vi "Main.vi"() -> ()   [LabVIEW 2018, in "MQTT_Singleton.lvlib"]
doc: "This template is based off of the Queued Message Handler design pattern and the Queued Message Handler project template that ships with LabVIEW.\n\nThe main difference is that the queue is private to this module and communication between modules is performed via Broadcast and Request events.\n\nRequest events are wrapped in public API methods and are handled in the Event Handling Loop (EHL) of this VI. Any module can register for Broadcast events sent by this module. The EHL generates messages based on user interface actions.\n\nThe Message Handling Loop (MHL) processes messages generated by the EHL, or by other messages. The messages are string values, so new messages can be added easily to the Message Cases case structure in the MHL. Each message cluster can also provide an optional value for Message Data, which is a variant that can be converted to whatever message-specific data is required.\n_____\nBased on Delacor QMH Project Template 4.1.0.59."
uses:
  MQTT_Singleton.lvlib
  <vilib>/Delacor/Delacor QMH/Libraries/Module Admin_class/Delacor_lib_QMH_Module Admin.lvclass
  Module Data--cluster.ctl
  LVMQTT-master/Controls/Connection_Return_Codes.ctl
  LVMQTT-master/Controls/QoS.ctl
  LVMQTT-master/Controls/DUP_Flag.ctl
  LVMQTT-master/Controls/Retain_Flag.ctl
  Stop Argument--cluster.ctl
  <vilib>/Delacor/Delacor QMH/Libraries/Module Admin_class/Delacor_lib_QMH_Module Admin.lvclass/Delacor_lib_QMH_Module Admin.ctl
  Connect Argument--cluster.ctl
  Publish Argument--cluster.ctl
  Subscribe Argument--cluster.ctl
  Disconnect Argument--cluster.ctl
  <vilib>/Utility/miscctls.llb/LVPointTypeDef.ctl
  LVMQTT-master/Controls/Connect_Flags.ctl
  <vilib>/Delacor/Delacor QMH/Libraries/Module Admin_class/Delacor_lib_QMH_Get External Launch.vi
  HB.vi
  <vilib>/Delacor/Delacor QMH/Libraries/Message Queue_class/Delacor_lib_QMH_Enqueue Message (Single).vi
  <vilib>/Utility/error.llb/Error Cluster From Error Code.vi
  <vilib>/ErrorRing/Error Ring.xnode
  <vilib>/Delacor/Delacor QMH/Libraries/Message Queue_class/Delacor_lib_QMH_Message Queue.lvclass
  LVMQTT-master/MQTT_Functions.lvlib
  MQTT Messages.lvlib
panel:
  out "Publish Message":string
  out "Publish Topic":string
  out "HB RX Count":u32
  out "Subscribe Topic":string
  out "Rx Message":string
  out "Rx Topic Name":string
  out "Latency (ms)":u32
  out "ms":u32
  out "HB TX Count":u32
  out "Acknowledged":bool
  out "error out":errorcluster
  in  "Module Admin":refnum<class "Delacor_lib_QMH_Module Admin.lvclass">
  out "Status":string
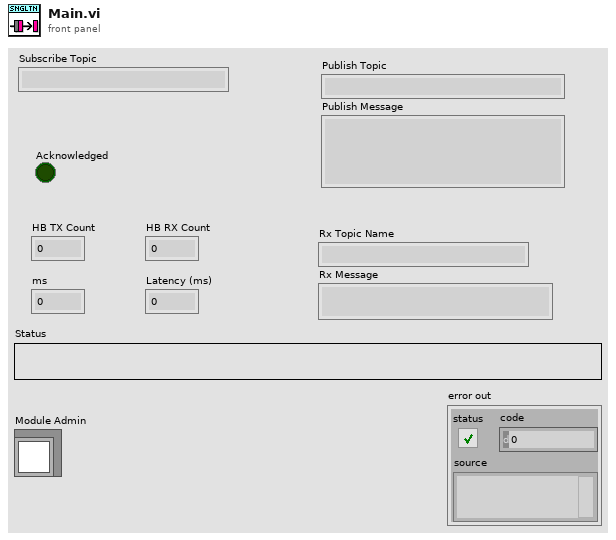
[diagram p1: front panel]
types:
  T1 = typedef "MQTT_Singleton.lvlib/Request Events--cluster.ctl" = cluster{"Stop Module":refnum<user-event>, "Show Panel":refnum<user-event>, "Hide Panel":refnum<user-event>, "Get Module Execution Status":refnum<user-event>, "Show Diagram":refnum<user-event>, "Connect":refnum<user-event>, "Publish":refnum<user-event>, "Subscribe":refnum<user-event>, "Disconnect":refnum<user-event>, "Start Listening":refnum<user-event>, "Stop Listening":refnum<user-event>, "Exit Listening":refnum<user-event>}
  T2 = typedef "MQTT_Singleton.lvlib/Module Data--cluster.ctl" = cluster{"Status":string, "connection ID out":refnum<k5>, "Connection Status":T3, "Connect Meta":cluster{"QoS":T4, "DUP":T5, "Retain":T6, "Keep Alive (sec)":u16}, "Message ID":u16, "Listening?":bool, "Default Topics":string[], "Broker IP":string, "Client ID":string}
  T3 = typedef "MQTT_Functions.lvlib/Connection_Return_Codes.ctl" = enum16{"Connection accepted", "Connection refused: unacceptable protocol version", "Connection refused: identifier rejected", "Connection refused: Server unavailable", "Connection refused: bad user name or password", "Connection refused: not authorized"}
  T4 = typedef "MQTT_Functions.lvlib/QoS.ctl" = enum8{"At most once", "At least once", "Exactly once", "Reserved"}
  T5 = typedef "MQTT_Functions.lvlib/DUP_Flag.ctl" = bool
  T6 = typedef "MQTT_Functions.lvlib/Retain_Flag.ctl" = bool
  T7 = enum32{"invalid lock state", "Not Locked", "Locked (No Password)", "Password-protected"}
  T8 = typedef "MQTT_Singleton.lvlib/Stop Argument--cluster.ctl" = cluster{"Origin":string, "Exit via Stop Module Req?":bool, "Wait for Module to stop?":bool}
  T9 = typedef "MQTT_Singleton.lvlib/Connect Argument--cluster.ctl" = cluster{"Broker IP":string, "ClientID":string}
  T10 = typedef "MQTT_Singleton.lvlib/Publish Argument--cluster.ctl" = cluster{"Topic":string, "Message":string}
  T11 = typedef "MQTT_Singleton.lvlib/Subscribe Argument--cluster.ctl" = cluster{"Topic":string}
  T12 = typedef "MQTT_Singleton.lvlib/Disconnect Argument--cluster.ctl" = cluster{"Disconnect?":bool}
  T13 = typedef "LVPointTypeDef.ctl" = cluster{"Horizontal":i16, "Vertical":i16}
  T14 = enum32{"Invalid", "Standard", "Closed", "Hidden", "Minimized", "Maximized"}
  T15 = cluster{"QoS":T4, "DUP":T5, "Retain":T6, "Keep Alive (sec)":u16}
  T16 = typedef "MQTT_Functions.lvlib/Connect_Flags.ctl" = cluster{"user name":bool, "password":bool, "will retain":bool, "will flag":bool, "clean session":bool, "reserved":bool, "will QoS":T4}
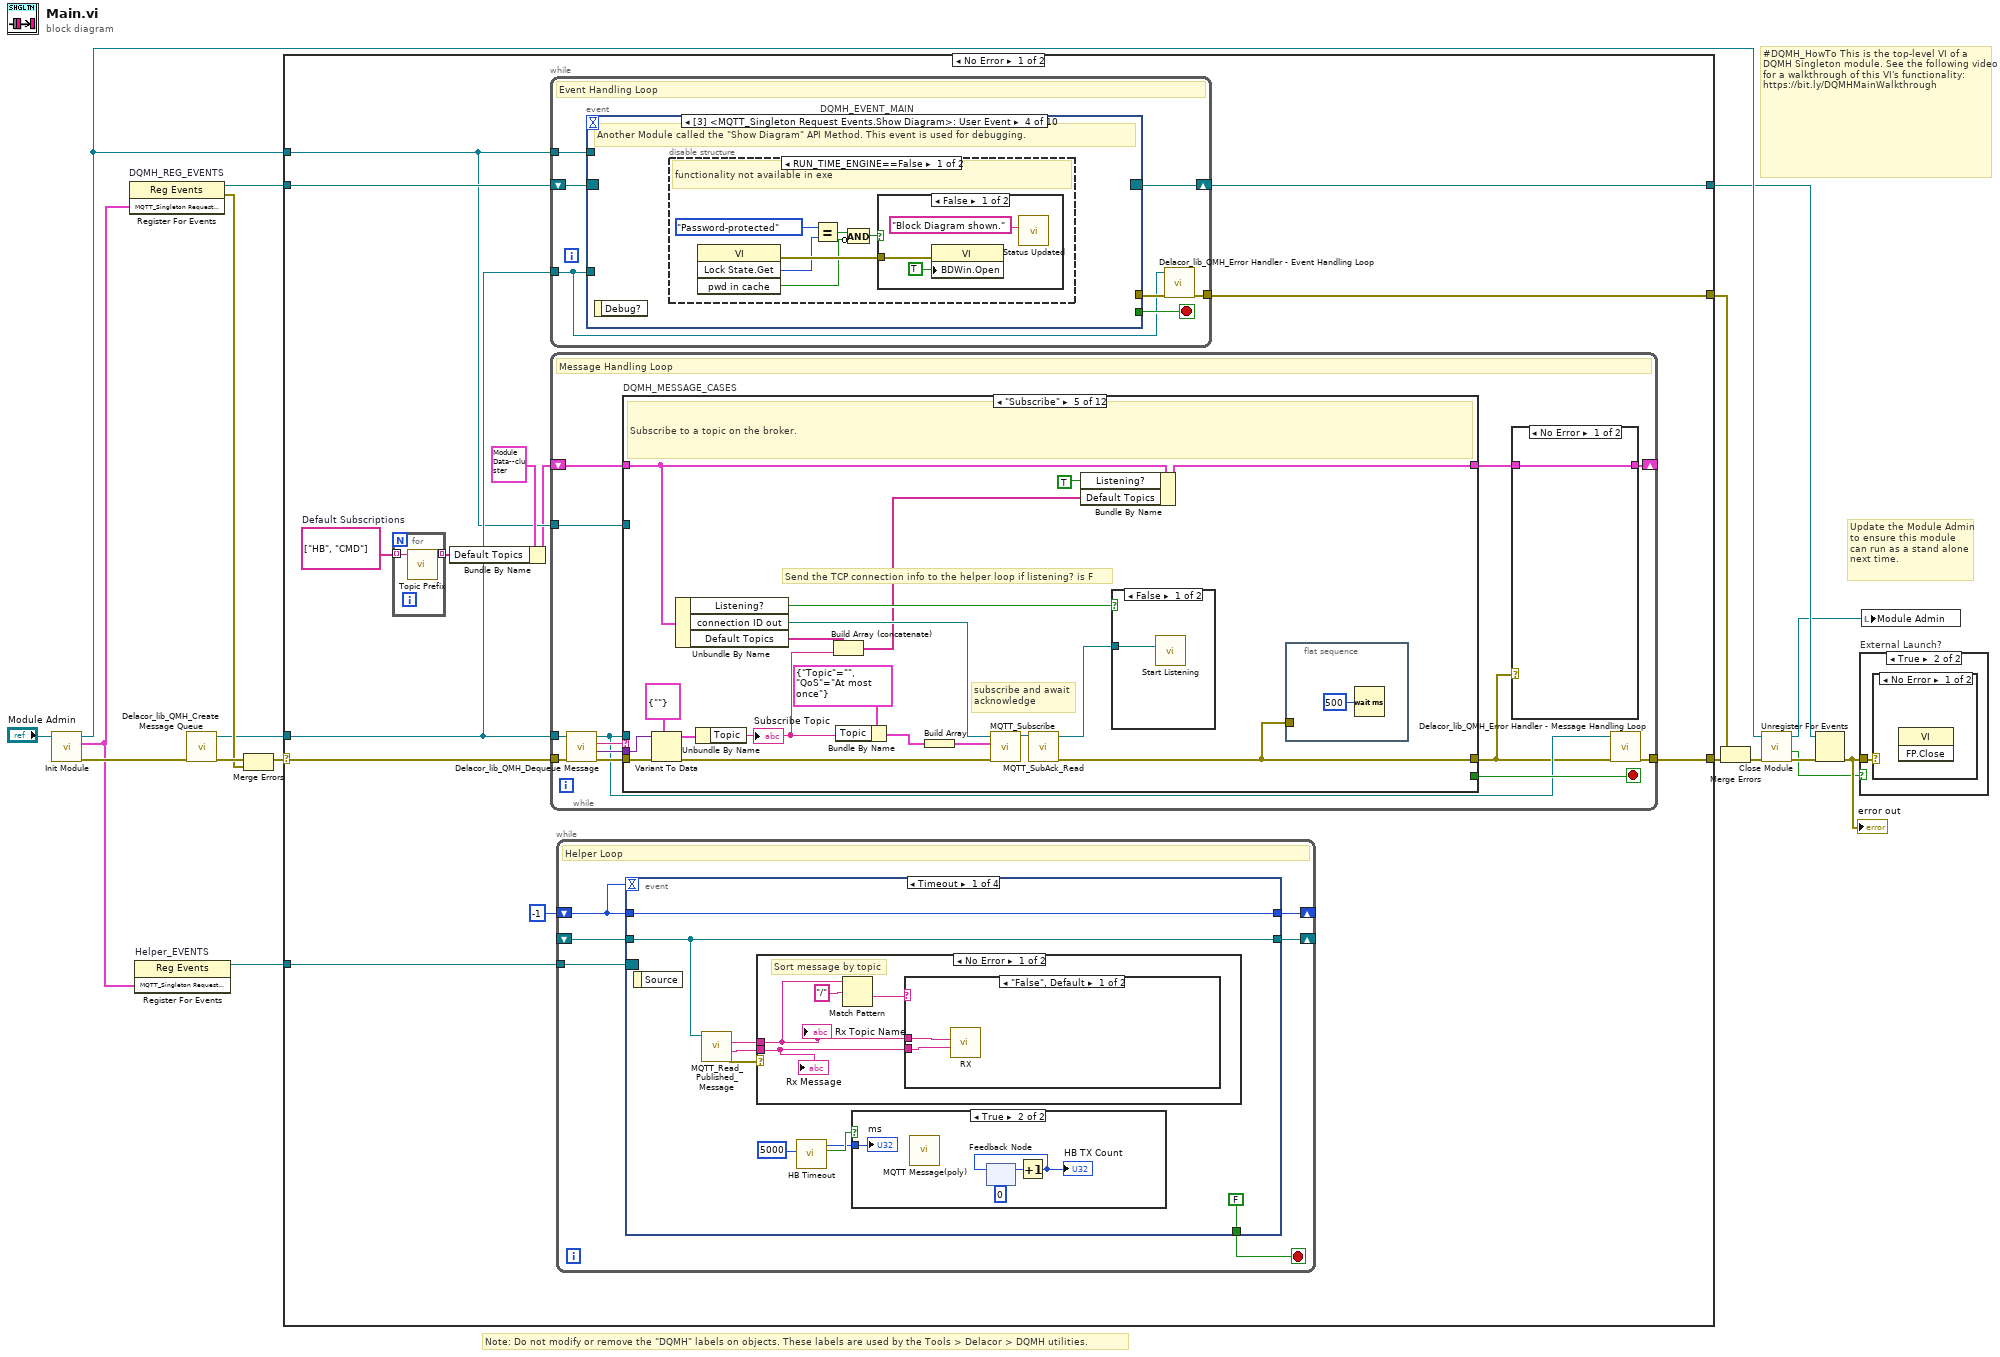
[diagram p0: block diagram]
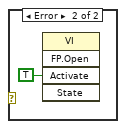
[diagram p3: hidden frame]
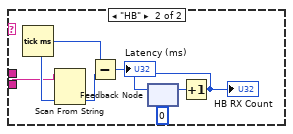
[diagram p5: hidden frame]
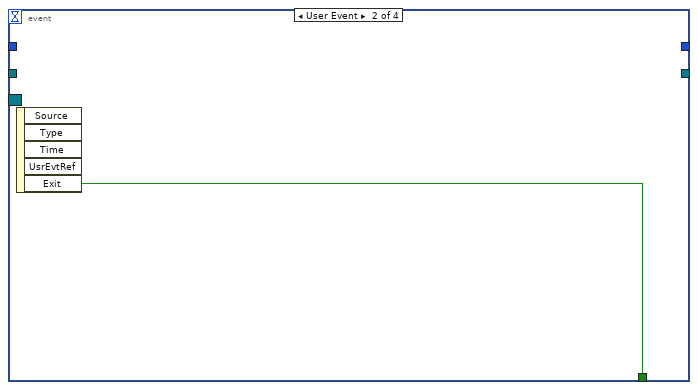
[diagram p7: hidden frame]
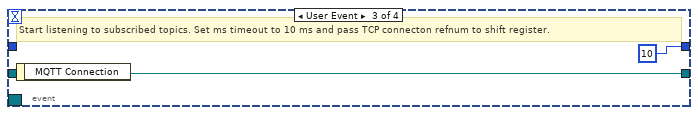
[diagram p8: hidden frame]
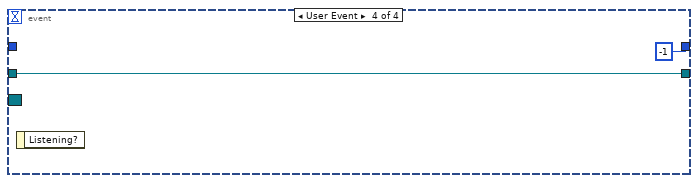
[diagram p9: hidden frame]
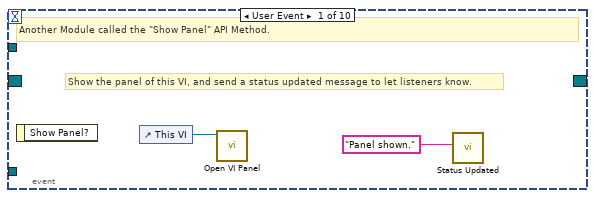
[diagram p10: hidden frame]
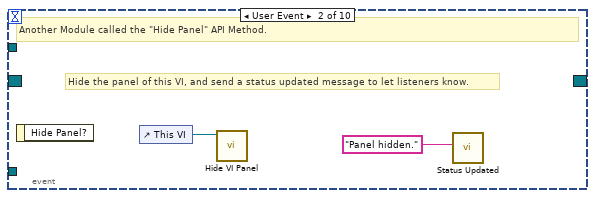
[diagram p11: hidden frame]
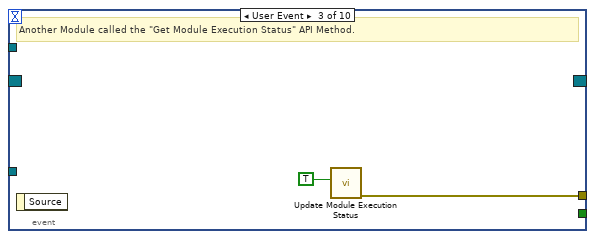
[diagram p12: hidden frame]
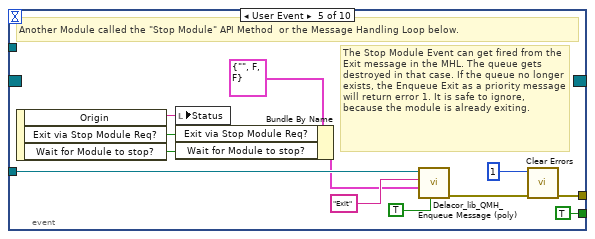
[diagram p15: hidden frame]
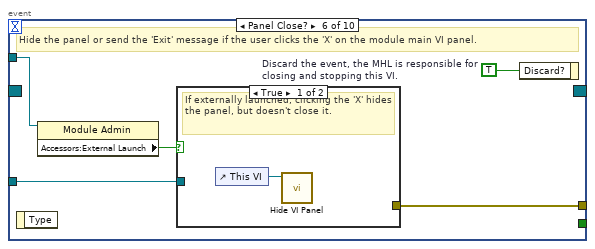
[diagram p16: hidden frame]
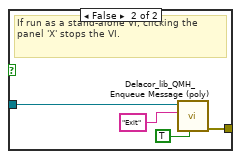
[diagram p17: hidden frame]
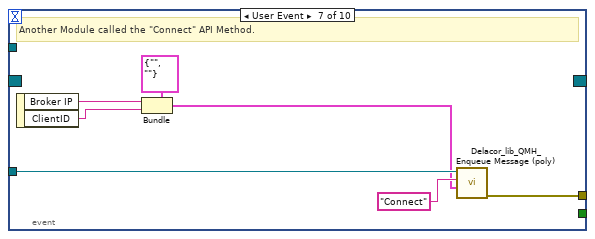
[diagram p18: hidden frame]
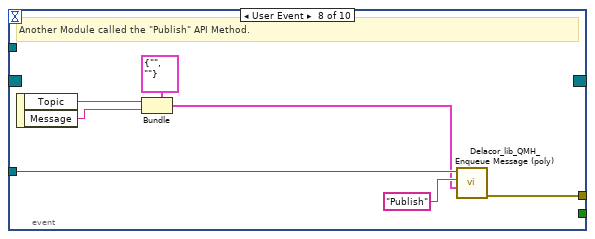
[diagram p19: hidden frame]
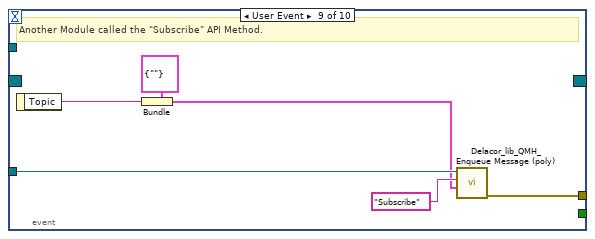
[diagram p20: hidden frame]
diagram:
  # "#DQMH_HowTo This is the top-level VI of a DQMH Singleton module. See the following video for a walkthrough of this VI's functionality: https://bit.ly/DQMHMainWalkthrough"
  # "Note: Do not modify or remove the \"DQMH\" labels on objects. These labels are used by the Tools > Delacor > DQMH utilities."
  # "Update the Module Admin to ensure this module can run as a stand alone next time."
  n1 = call "Init Module.vi"("Singleton Module Admin in"="Module Admin") -> ("error out"=w17:errorcluster, "MQTT_Singleton Request Events"=w2:T1, "Singleton Module Admin out"=w9:refnum<class "Delacor_lib_QMH_Module Admin.lvclass">)  [unwired: 8 in]
  n2 = register-events "DQMH_REG_EVENTS"(w2) -> (reference out=w7:refnum<event-registration>, error out=w10:errorcluster)  [unwired: 2 in]
  n3 = register-events "Helper_EVENTS"(w2) -> (reference out=w1:refnum<event-registration>)  [unwired: 2 in, 1 out]
  n4 = call <vilib>:"Delacor_lib_QMH_Create Message Queue.vi"("error in (no error)"=w17) -> ("error out"=w12:errorcluster, "Message Queue"=w6:refnum<class "Delacor_lib_QMH_Message Queue.lvclass">)  [unwired: 9 in]
  n5 = Merge Errors(w12, w10) -> (w11:errorcluster)
  n6 = case shown="No Error" w11 {
    selector: w11 -> [w29 w371]
    tunnel: [w31 w371] -> w18
    tunnel: [w28 w368] -> w8
    tunnel: w7 -> [w26 w368]
    tunnel: w6 -> [w25 _]
    tunnel: [w30 _] -> w15
    tunnel: w9 -> [w24 w364]
    tunnel: w1 -> [w22 _]
    frame No Error {
      w20 = string[] ["HB", "CMD"]  # Default Subscriptions
      n7 = for {
        tunnel: w20 -> [w33] mode=indexing
        tunnel: [w32] -> w19 mode=indexing
        n8 = call "Topic Prefix.vi"("Topic"=w33) -> ("Topic"=w32:string)  [unwired: 9 in, 1 out]
      }
      n9 = Bundle By Name(cluster=T2 {"Status"="", "connection ID out"=refnum, "Connection Status"=enum."Connection refused: not authorized", "Connect Meta"={"QoS"=enum."At most once", "DUP"=FALSE, "Retain"=FALSE, "Keep Alive (sec)"=60}, "Message ID"=10, "Listening?"=FALSE, "Default Topics"=[], "Broker IP"="", "Client ID"=""} ("Data Cluster"), "Default Topics"=w19) -> (w21:T2)
      n10 = while {
        tunnel: w25 -> [w71]
        shift-right: [w74] -> w28
        shift-left: w26 -> [w75]
        tunnel: [w76] -> w30
        tunnel: w24 -> [w72]
        stop <- w73 stop-if-true
        # "Event Handling Loop"
        n11 = event "DQMH_EVENT_MAIN" shown="[3] <MQTT_Singleton Request Events.Show Diagram>: User Event" {
          selector: w75 -> [_ _ _ _ _ _ _ _ _ _]
          dyn-events: [_ _ _ _ _ _ _ _ _ _] -> w74
          timeout: _ -> [_ _ _ _ _ _ _ _ _ _]
          tunnel: [_ _ _ _ TRUE ("Discard?") _ _ _ _ _] -> w73
          tunnel: w71 -> [_ _ _ _ w100 w107 w121 w128 w134 w140]
          tunnel: [_ _ w83 _ w103 w109 w115 w122 w129 w135] -> w77
          tunnel: w72 -> [_ _ _ _ _ w106 _ _ _ _]
          event User Event {
            # "Show the panel of this VI, and send a status updated message to let listeners know."
            # "Another Module called the \"Show Panel\" API Method."
            n12 = event-data() -> ()  [unwired: 1 in, 1 out]
            n13 = control-ref of="This VI"() -> (w79:refnum<vi>)
            n14 = call "Open VI Panel.vi"("VI"=w79) -> ()  [unwired: 10 in, 1 out]
            n15 = call "Status Updated.vi"("Status"="Panel shown." ("format string")) -> ()  [unwired: 10 in, 1 out]
          }
          event User Event {
            # "Hide the panel of this VI, and send a status updated message to let listeners know."
            # "Another Module called the \"Hide Panel\" API Method."
            n16 = event-data() -> ()  [unwired: 1 in, 1 out]
            n17 = control-ref of="This VI"() -> (w81:refnum<vi>)
            n18 = call "Hide VI Panel.vi"("VI"=w81) -> ()  [unwired: 10 in, 1 out]
            n19 = call "Status Updated.vi"("Status"="Panel hidden." ("format string")) -> ()  [unwired: 10 in, 1 out]
          }
          event User Event {
            # "Another Module called the \"Get Module Execution Status\" API Method."
            n20 = event-data() -> ()  [unwired: 1 in, 1 out]
            n21 = call "Update Module Execution Status.vi"("Running?"=TRUE) -> ("error out"=w83:errorcluster)  [unwired: 10 in]
          }
          event User Event {
            # "Another Module called the \"Show Diagram\" API Method. This event is used for debugging."
            n22 = event-data() -> ()  [unwired: 1 in, 1 out]
            n23 = disable-structure shown="RUN_TIME_ENGINE==False" {
              frame condition #0 (active) {
                # "functionality not available in exe"
                n24 = invoke class="VI" method="Lock State.Get"() -> (error out=w89:errorcluster, "Get Lock State"=w88:T7, "pwd in cache"=w85:bool)  [unwired: 4 in, 1 out]
                n25 = Equal?(x=T7."Password-protected", y=w88) -> (x = y?=w86:bool)
                n26 = Compound Arithmetic op=AND(w86, invert w85) -> (w84:bool)
                n27 = case shown="False" w84 {
                  tunnel: w89 -> [w92 _]
                  frame False {
                    n28 = property class="VI"(error in=w92, "BDWin.Open"=TRUE ("Block Diagram Window:Open")) -> ()  [unwired: 1 in, 2 out]
                    n29 = call "Status Updated.vi"("Status"="Block Diagram shown." ("format string")) -> ()  [unwired: 10 in, 1 out]
                  }
                  frame True {
                    # "Password-protected VI, and the password is not in the cache. Do not show the diagram."
                  }
                }
              }
              frame condition #1 {
              }
            }
          }
          event User Event {
            # "The Stop Module Event can get fired from the Exit message in the MHL. The queue gets destroyed in that case. If the queue no longer exists, the Enqueue Exit as a priority message will return error 1. It is safe to ignore, because the module is already exiting."
            # "Another Module called the \"Stop Module\" API Method  or the Message Handling Loop below."
            n30 = event-data() -> ("Origin"=w99:string, "Exit via Stop Module Req?"=w95:bool, "Wait for Module to stop?"=w94:bool)  [unwired: 1 in]
            n31 = local write "Status"(w99) -> ()
            n32 = Bundle By Name(cluster=T8 {"Origin"="", "Exit via Stop Module Req?"=FALSE, "Wait for Module to stop?"=FALSE} ("Stop Argument"), "Exit via Stop Module Req?"=w95, "Wait for Module to stop?"=w94) -> (w93:T8)
            n33 = call-poly <vilib>:"Delacor_lib_QMH_Enqueue Message (poly).vi"("Priority Message? (F)"=TRUE, "Message Data"=w93, "Message"="Exit", "Message Queue in"=w100) -> ("error out"=w104:errorcluster)  [unwired: 6 in, 1 out]
            n34 = call <vilib>:"Clear Errors.vi"("error in (no error)"=w104, "specific error code to clear (0: all)"=1) -> ("error out"=w103:errorcluster)  [unwired: 4 in, 1 out]
          }
          event Panel Close? {
            w108 = TRUE  # Discard the event, the MHL is responsible for closing and stopping this VI.
            # "Hide the panel or send the 'Exit' message if the user clicks the 'X' on the module main VI panel."
            n35 = event-data() -> ()  [unwired: 1 in, 1 out]
            n36 = property class="Module Admin"(reference=w106) -> ("Accessors:External Launch"=w105:bool)  [unwired: 1 in, 2 out]
            n37 = case shown="True" w105 {
              tunnel: w107 -> [_ w113]
              tunnel: [_ w114] -> w109
              frame True {
                # "If externally launched, clicking the 'X' hides the panel, but doesn't close it."
                n38 = control-ref of="This VI"() -> (w110:refnum<vi>)
                n39 = call "Hide VI Panel.vi"("VI"=w110) -> ()  [unwired: 10 in, 1 out]
              }
              frame False {
                # "If run as a stand-alone VI, clicking the panel 'X' stops the VI."
                n40 = call-poly <vilib>:"Delacor_lib_QMH_Enqueue Message (poly).vi"("Priority Message? (F)"=TRUE, "Message"="Exit", "Message Queue in"=w113) -> ("error out"=w114:errorcluster)  [unwired: 7 in, 1 out]
              }
            }
            n41 = event-data("Discard?"=w108) -> ()  [unwired: 1 in, 1 out]
          }
          event User Event {
            # "Another Module called the \"Connect\" API Method."
            n42 = event-data() -> ("Broker IP"=w117:string, "ClientID"=w116:string)  [unwired: 1 in]
            n43 = Bundle(cluster=T9 {"Broker IP"="", "ClientID"=""} ("Connect Argument"), "Broker IP"=w117, "ClientID"=w116) -> (w118:T9)
            n44 = call-poly <vilib>:"Delacor_lib_QMH_Enqueue Message (poly).vi"("Message Data"=w118, "Message"="Connect", "Message Queue in"=w121) -> ("error out"=w115:errorcluster)  [unwired: 7 in, 1 out]
          }
          event User Event {
            # "Another Module called the \"Publish\" API Method."
            n45 = event-data() -> ("Topic"=w124:string, "Message"=w123:string)  [unwired: 1 in]
            n46 = Bundle(cluster=T10 {"Topic"="", "Message"=""} ("Publish Argument"), "Topic"=w124, "Message"=w123) -> (w125:T10)
            n47 = call-poly <vilib>:"Delacor_lib_QMH_Enqueue Message (poly).vi"("Message Data"=w125, "Message"="Publish", "Message Queue in"=w128) -> ("error out"=w122:errorcluster)  [unwired: 7 in, 1 out]
          }
          event User Event {
            # "Another Module called the \"Subscribe\" API Method."
            n48 = event-data() -> ("Topic"=w130:string)  [unwired: 1 in]
            n49 = Bundle(cluster=T11 {"Topic"=""} ("Subscribe Argument"), "Topic"=w130) -> (w131:T11)
            n50 = call-poly <vilib>:"Delacor_lib_QMH_Enqueue Message (poly).vi"("Message Data"=w131, "Message"="Subscribe", "Message Queue in"=w134) -> ("error out"=w129:errorcluster)  [unwired: 7 in, 1 out]
          }
          event User Event {
            # "Another Module called the \"Disconnect\" API Method."
            n51 = event-data() -> ("Disconnect?"=w136:bool)  [unwired: 1 in]
            n52 = Bundle(cluster=T12 {"Disconnect?"=FALSE} ("Disconnect Argument"), "Disconnect?"=w136) -> (w137:T12)
            n53 = call-poly <vilib>:"Delacor_lib_QMH_Enqueue Message (poly).vi"("Message Data"=w137, "Message"="Disconnect", "Message Queue in"=w140) -> ("error out"=w135:errorcluster)  [unwired: 7 in, 1 out]
          }
        }
        n54 = call-dynamic "Delacor_lib_QMH_Error Handler - Event Handling Loop.vi"("error in (no error)"=w77, "Message Queue in"=w71) -> ("dup error in"=w76:errorcluster)  [unwired: 8 in, 1 out]
      }
      n55 = while {
        tunnel: w25 -> [w146]
        shift-right: [w142] -> _
        shift-left: w21 -> [w150]
        tunnel: w29 -> [w153]
        tunnel: [w151] -> w31
        tunnel: w24 -> [w144]
        stop <- w149 stop-if-true
        # "Message Handling Loop"
        n56 = call-dynamic "Delacor_lib_QMH_Dequeue Message.vi"("error in (no error)"=w153, "Message Queue in"=w146) -> ("error out"=w152:errorcluster, "Message Data"=w147:variant, "Message"=w148:string, "Message Queue out"=w145:refnum<class "Delacor_lib_QMH_Message Queue.lvclass">)  [unwired: 6 in]
        n57 = case "DQMH_MESSAGE_CASES" shown="\"Subscribe\"" w148 {
          selector: w148 -> [_ _ _ _ _ _ _ _ _ _ _ w351]
          tunnel: w145 -> [_ _ _ _ _ _ _ _ _ w319 w344 _]
          tunnel: w152 -> [w178 w182 w206 w242 w284 w298 w302 w304 w309 w326 w349 w353]
          tunnel: [w176 w182 w192 w225 w269 w288 w301 w304 w308 w322 w334 w354] -> w143
          tunnel: w150 -> [w167 w181 w205 w238 w280 w295 w300 w303 w306 w321 w343 w352]
          tunnel: [w166 w181 w183 w238 w271 w291 w300 w303 w306 w321 w343 w352] -> w141
          tunnel: [_ _ _ _ _ _ _ _ _ _ w336 _] -> w149
          tunnel: w147 -> [_ _ w204 w241 w283 w297 _ _ _ w320 w342 _]
          tunnel: w144 -> [w168 _ _ _ _ _ _ _ _ w318 w337 _]
          frame "Initialize" {
            w161 = "Initial Message" ("Initial Message")
            # "#CodeNeeded - Initialize the appearance of the front panel."
            # "#CodeNeeded - Initialize your state data here."
            # "Initialize - Any operation that needs to be done before the module can receive messages. Synchronize Caller Events.vi will inform Start Module.vi that the module has launched and is ready to receive messages. Module Did Init.vi will broadcast that the module initialized."
            n58 = call "Synchronize Caller Events.vi"("error in (no error)"=w178, "Singleton Module Admin in"=w168) -> ("error out"=w177:errorcluster, "Singleton Module Admin out"=w163:refnum<class "Delacor_lib_QMH_Module Admin.lvclass">)  [unwired: 8 in]
            n59 = property class="Module Admin"(reference=w163) -> ("Accessors:External Launch"=w172:bool)  [unwired: 1 in, 2 out]
            n60 = Select(t=T14."Hidden" ("State"), s=w172, f=T14."Standard" ("State")) -> (s? t:f=w169:T14)
            n61 = call "Module Name--constant.vi"() -> ("Module Name"=w175:string)  [unwired: 11 in]
            n62 = property class="VI"("Front Panel.Title"=w175) -> (reference out=w174:refnum<vi>, error out=w180:errorcluster)  [unwired: 2 in]
            n63 = call "Module Name--constant.vi"() -> ("Module Name"=w164:string)  [unwired: 11 in]
            n64 = invoke class="VI" method="FP.Open"(reference=w174, error in=w180, "State"=w169) -> (reference out=w173:refnum<vi>, error out=w179:errorcluster)  [unwired: 2 in, 3 out]
            n65 = Bundle By Name(cluster=w167, "Status"=w161) -> (w166:T2)
            n66 = call "Module Did Init.vi"("error in (no error)"=w177, "Initialized?"=TRUE, "Origin"=w164) -> ("error out"=w176:errorcluster)  [unwired: 8 in]
            n67 = invoke class="VI" method="FP.Center"(reference=w173, error in=w179) -> ()  [unwired: 1 in, 3 out]
            n68 = property on="Pane" class="Pane"("Origin"=T13 {"Horizontal"=0, "Vertical"=0}) -> ()  [unwired: 2 in, 2 out]
            "Status" <- w161
          }
          frame "--- Module Specific ---" {
            # "Separator -- The following cases handle messages specific to this Module."
          }
          frame "Connect" {
            w195 = T15 {"QoS"=enum."At most once", "DUP"=FALSE, "Retain"=FALSE, "Keep Alive (sec)"=60}  # Connect Meta
            w201 = T16 {"user name"=FALSE, "password"=FALSE, "will retain"=FALSE, "will flag"=FALSE, "clean session"=FALSE, "reserved"=FALSE, "will QoS"=enum."At most once"}  # Connect Flags
            # "Connect to Broker"
            n69 = Variant To Data(error in=w206, type=T9 {"Broker IP"="", "ClientID"=""} ("Connect Argument"), Variant=w204) -> (data=w202:T9, error out=w198:errorcluster)
            n70 = Unbundle By Name(w202) -> ("Broker IP"=w185:string, "ClientID"=w184:string)
            n71 = Bundle By Name(cluster=cluster{"address (IP)":string, "port":u16} {"address (IP)"="", "port"=1883} ("MQTT Broker"), "address (IP)"=w185) -> (w199:cluster{"address (IP)":string, "port":u16})
            n72 = Bundle By Name(cluster=w201, "clean session"=TRUE) -> (w191:T16)
            n73 = call "MQTT_Connect.vi"("Connect Meta"=w195, "Client ID"=w184, "Connect Flags"=w191, "error in (no error)"=w198, "MQTT Broker"=w199) -> ("error out"=w189:errorcluster, "Connection Status"=w193:T3, "connection ID out"=w197:refnum<k5>)  [unwired: 4 in]
            n74 = Format Into String(w193) -> (resulting string=w196:string)  [unwired: 3 in, 1 out]
            n75 = Bundle By Name(cluster=w205, "Broker IP"=w185, "Client ID"=w184, "Status"=w196, "connection ID out"=w197, "Connection Status"=w193, "Connect Meta"=w195) -> (w186:T2)
            n76 = Equal?(x=w193, y=Connection_Return_Codes."Connection accepted" ("Connection Status")) -> (x = y?=w188:bool)
            n77 = call "Connection Status.vi"("error in (no error)"=w189, "Connection OK?"=w188) -> ("error out"=w187:errorcluster)  [unwired: 9 in]
            n78 = case shown="True" w188 {
              tunnel: [w208 w215] -> w192
              tunnel: w187 -> [w208 w217]
              tunnel: w186 -> [w207 w212]
              tunnel: [w207 w211] -> w183
              frame False {
              }
              frame True {
                # "Always subscribe to default topics"
                # "subscribe and await\nacknowledge"
                n79 = Unbundle By Name(w212) -> ("connection ID out"=w214:refnum<k5>, "Default Topics"=w218:string[])
                n80 = for {
                  tunnel: w218 -> [w223] mode=indexing
                  tunnel: [w222] -> w216 mode=indexing
                  n81 = Bundle By Name(cluster=cluster{"Topic":string, "QoS":T4} {"Topic"="", "QoS"=enum."At most once"} ("Subscription Info"), "Topic"=w223) -> (w222:cluster{"Topic":string, "QoS":T4})
                }
                n82 = call "MQTT_Subscribe.vi"("error in (no error)"=w217, "Subscription Info Array"=w216, "connection ID"=w214) -> ("connection ID out"=w219:refnum<k5>)  [unwired: 7 in, 1 out]
                n83 = Bundle By Name(cluster=w212, "Listening?"=TRUE) -> (w211:T2)
                n84 = call "MQTT_SubAck_Read.vi"("connection ID"=w219) -> ("error out"=w215:errorcluster, "connection ID out"=w213:refnum<k5>)  [unwired: 8 in, 1 out]
                n85 = flat-sequence {
                  tunnel: w213 -> [w221]
                  tunnel: u32 1000 ("milliseconds to wait") -> [w220]
                  frame #0 {
                    n86 = call "Start Listening.vi"("MQTT Connection"=w221) -> ()  [unwired: 10 in, 1 out]
                    n87 = Wait (ms)(milliseconds to wait=w220) -> ()  [unwired: 1 out]
                  }
                }
              }
            }
          }
          frame "Publish" {
            # "Publish a message to the broker on a specific topic"
            n88 = Variant To Data(error in=w242, type=T10 {"Topic"="", "Message"=""} ("Publish Argument"), Variant=w241) -> (data=w239:T10, error out=w226:errorcluster)
            n89 = Unbundle By Name(w238) -> ("Connect Meta"=w234:T15, "connection ID out"=w233:refnum<k5>)
            n90 = Unbundle By Name(w239) -> ("Topic"=w232:string, "Message"=w231:string)
            "Publish Topic" <- w232
            "Publish Message" <- w231
            n91 = Unbundle By Name(w234) -> ("QoS"=w237:T4)
            n92 = feedback #1() -> (w229:u16)  [unwired: 1 in]
            n93 = Increment(x=w229) -> (x+1=w228:u16)
            n94 = call "MQTT_Publish.vi"("Message ID"=w228, "error in (no error)"=w226, "Message to be published"=w231, "Topic"=w232, "connection ID"=w233) -> ("error out"=w236:errorcluster, "connection ID out"=w235:refnum<k5>)  [unwired: 5 in]
            n95 = case shown="\"At most once\", Default" w237 {
              tunnel: w236 -> [w245 w252 w264]
              tunnel: w235 -> [w246 w253 w265]
              tunnel: [w245 w250 w257] -> w225
              tunnel: [w246 w249 w258] -> _
              tunnel: w228 -> [w243 w251 w263]
              tunnel: [FALSE w248 w259] -> w227
              tunnel: [w243 w247 w256] -> w230
              frame "At most once", Default {
                # "QoS 0: no PubACK, fire and forget"
              }
              frame "At least once" {
                # "QoS 1: PubACK"
                n96 = call "MQTT_PubAck_Read.vi"("error in (no error)"=w252, "connection ID"=w253) -> ("error out"=w250:errorcluster, "Message ID"=w247:u16, "connection ID out"=w249:refnum<k5>)  [unwired: 7 in]
                n97 = Equal?(x=w247, y=w251) -> (x = y?=w248:bool)
              }
              frame "Exactly once" {
                # "QoS 2: PubREC, PubREL, PubCOMP"
                n98 = call "MQTT_PubRec_Read.vi"("error in (no error)"=w264, "connection ID"=w265) -> ("error out"=w262:errorcluster, "Message ID"=w260:u16, "connection ID out"=w261:refnum<k5>)  [unwired: 7 in]
                n99 = call "MQTT_PubRel_Send.vi"("error in (no error)"=w262, "Message ID"=w260, "connection ID"=w261) -> ("error out"=w254:errorcluster, "connection ID out"=w255:refnum<k5>)  [unwired: 6 in, 1 out]
                n100 = call "MQTT_PubComp_Read.vi"("error in (no error)"=w254, "connection ID"=w255) -> ("error out"=w257:errorcluster, "Message ID"=w256:u16, "connection ID out"=w258:refnum<k5>)  [unwired: 7 in]
                n101 = Equal?(x=w256, y=w263) -> (x = y?=w259:bool)
              }
            }
            "Acknowledged" <- w227
            n102 = feedback-in #1(w230) -> ()
          }
          frame "Subscribe" {
            # "Send the TCP connection info to the helper loop if listening? is F"
            # "subscribe and await\nacknowledge"
            # "Subscribe to a topic on the broker."
            n103 = Variant To Data(error in=w284, type=T11 {"Topic"=""} ("Subscribe Argument"), Variant=w283) -> (data=w281:T11, error out=w277:errorcluster)
            n104 = Unbundle By Name(w280) -> ("Listening?"=w272:bool, "connection ID out"=w278:refnum<k5>, "Default Topics"=w268:string[])
            n105 = Unbundle By Name(w281) -> ("Topic"=w267:string)
            "Subscribe Topic" <- w267
            n106 = Build Array (concatenate)(w268, w267) -> (w266:string[])
            n107 = Bundle By Name(cluster=cluster{"Topic":string, "QoS":T4} {"Topic"="", "QoS"=enum."At most once"} ("Subscription Info"), "Topic"=w267) -> (w274:cluster{"Topic":string, "QoS":T4})
            n108 = Build Array(w274) -> (w273:cluster{"Topic":string, "QoS":T4}[])
            n109 = call "MQTT_Subscribe.vi"("error in (no error)"=w277, "Subscription Info Array"=w273, "connection ID"=w278) -> ("connection ID out"=w279:refnum<k5>)  [unwired: 7 in, 1 out]
            n110 = call "MQTT_SubAck_Read.vi"("connection ID"=w279) -> ("error out"=w269:errorcluster, "connection ID out"=w276:refnum<k5>)  [unwired: 8 in, 1 out]
            n111 = Bundle By Name(cluster=w280, "Listening?"=TRUE, "Default Topics"=w266) -> (w271:T2)
            n112 = case shown="False" w272 {
              tunnel: w276 -> [w286 _]
              frame False {
                n113 = call "Start Listening.vi"("MQTT Connection"=w286) -> ()  [unwired: 10 in, 1 out]
              }
              frame True {
              }
            }
            n114 = flat-sequence {
              tunnel: w269 -> [_]
              frame #0 {
                n115 = Wait (ms)(milliseconds to wait=u32 500) -> ()  [unwired: 1 out]
              }
            }
          }
          frame "Disconnect" {
            # "Disconnect from the broker."
            n116 = Variant To Data(error in=w298, type=T12 {"Disconnect?"=FALSE} ("Disconnect Argument"), Variant=w297) -> (error out=w293:errorcluster)  [unwired: 1 out]
            n117 = Unbundle By Name(w295) -> ("Listening?"=w292:bool, "connection ID out"=w294:refnum<k5>)
            n118 = call "MQTT_Disconnect.vi"("error in (no error)"=w293, "connection ID"=w294) -> ("error out"=w289:errorcluster)  [unwired: 9 in]
            n119 = case shown="True" w292 {
              selector: w292 -> [_ w299]
              frame False {
              }
              frame True {
                n120 = call "Stop Listening.vi"("Listening?"=w299) -> ()  [unwired: 10 in, 1 out]
              }
            }
            n121 = Bundle By Name(cluster=w295, "Listening?"=FALSE) -> (w291:T2)
            n122 = call "Connection Status.vi"("error in (no error)"=w289, "Connection OK?"=FALSE) -> ("error out"=w288:errorcluster)  [unwired: 9 in]
          }
          frame "---Copy This Frame---" {
            # "Duplicate this frame when creating new messages.  Change this comment in the duplicated frame to describe this message."
            n123 = Merge Errors(w302) -> (w301:errorcluster)
          }
          frame "--- Exit and Error Handling---" {
            # "Separator - The following cases handle errors and exit messages."
          }
          frame "Simulate MHL Error" {
            # "#DQMH_HowTo The 'Simulate MHL Error' button  illustrates how the MHL handles errors. This event is instructional in nature and can be removed."
            # "Simulate an error occurring at the MHL"
            n124 = call "Module Name--constant.vi"() -> ("Module Name"=w305:string)  [unwired: 11 in]
            n125 = xnode "Error Ring"("parameter 0"=w305) -> ("error out"=w307:errorcluster)
            n126 = Merge Errors(w309, w307) -> (w308:errorcluster)
          }
          frame "Error" {
            # "#CodeRecommended - If you ever change the name of this \"Error\" message, you'll need to update the name in the Check Loop Error.vi as well."
            # "#CodeRecommended - If the module is running in standalone mode (External Launch = FALSE), this code will pop up an error dialog and call the 'Exit' message if an error occurs. Add more fine-grained error handling here."
            # "Error - Check the error message data and respond accordingly. This message is sent by the \"Error Handler\" VIs at the end of each loop in this application."
            n127 = property class="Module Admin"(reference=w318) -> ("Accessors:External Launch"=w317:bool)  [unwired: 1 in, 2 out]
            n128 = Variant To Data(error in=w326, type=errorcluster {"status"=FALSE, "code"=0, "source"=""} ("error constant"), Variant=w320) -> (data=w327:errorcluster, error out=w324:errorcluster)
            n129 = call "Error Reported.vi"("Error"=w327) -> ()  [unwired: 10 in, 1 out]
            n130 = case shown="False" w317 {
              tunnel: [w332 _] -> w323
              tunnel: w319 -> [w330 _]
              tunnel: w327 -> [w331 _]
              frame False {
                # "If the module is running standalone, then pop up an error dialog and call the \"Exit\" message."
                n131 = call <vilib>:"Simple Error Handler.vi"("error in (no error)"=w331) -> ()  [unwired: 4 in, 5 out]
                n132 = call-poly <vilib>:"Delacor_lib_QMH_Enqueue Message (poly).vi"("Priority Message? (F)"=TRUE, "Message"="Exit", "Message Queue in"=w330) -> ("error out"=w332:errorcluster)  [unwired: 7 in, 1 out]
              }
              frame True {
                # "If the module was launched externally, calling the Error Reported broadcast VI is the only action performed by the \"Error\" message. The module's caller can then process the error appropriately."
              }
            }
            n133 = Merge Errors(w324, w323) -> (w322:errorcluster)
            n134 = local write "error out"(w322) -> ()
          }
          frame "Exit" {
            w341 = 91  # 91: not all Exit messages will have an argument
            w336 = TRUE  # Stop the VI
            # "Release the message queue reference"
            # "#CodeNeeded - Add any required cleanup code here"
            # "Exit - Exit the application."
            n135 = Variant To Data(error in=w349, type=T8 {"Origin"="", "Exit via Stop Module Req?"=FALSE, "Wait for Module to stop?"=FALSE} ("Stop Argument"), Variant=w342) -> (data=w339:T8, error out=w346:errorcluster)
            n136 = call <vilib>:"Clear Errors.vi"("error in (no error)"=w346, "specific error code to clear (0: all)"=w341) -> ("error out"=w348:errorcluster)  [unwired: 4 in, 1 out]
            n137 = control-ref of="This VI"() -> (w338:refnum<vi>)
            n138 = call-dynamic "Delacor_lib_QMH_Release Message Queue.vi"("error in (no error)"=w348, "Message Queue"=w344) -> ("error out"=w347:errorcluster)  [unwired: 9 in]
            n139 = call "Handle Exit.vi"("Stop Argument"=w339, "Admin in"=w337, "VI reference"=w338) -> ("error out"=w345:errorcluster)  [unwired: 7 in, 1 out]
            n140 = Merge Errors(w347, w345) -> (w335:errorcluster)
            n141 = call "Connection Status.vi"("error in (no error)"=w335, "Connection OK?"=FALSE) -> ("error out"=w334:errorcluster)  [unwired: 9 in]
            n142 = call "Exit Listening.vi"("Exit"=w336) -> ()  [unwired: 10 in, 1 out]
          }
          frame Default {
            # "'Default' case only runs if there is a message that isn't defined in any of the other cases.  Output a programming error."
            n143 = call "Module Name--constant.vi"() -> ("Module Name"=w350:string)  [unwired: 11 in]
            n144 = xnode "Error Ring"("parameter 0"=w351, "parameter 1"=w350) -> ("error out"=w355:errorcluster)
            n145 = Merge Errors(w353, w355) -> (w354:errorcluster)
          }
        }
        n146 = case shown="No Error" w143 {
          tunnel: [w154 w159] -> w142
          tunnel: w141 -> [w154 w159]
          frame No Error {
          }
          frame Error {
            # "Disconnect &\nReconnect on error"
            n147 = Unbundle By Name(w159) -> ("Broker IP"=w158:string, "Client ID"=w157:string)
            n148 = call "Disconnect.vi"("Disconnect?"=TRUE) -> ("error out"=w160:errorcluster)  [unwired: 10 in]
            n149 = Wait (ms)(milliseconds to wait=u32 1000) -> ()  [unwired: 1 out]
            n150 = call "Connect.vi"("error in (no error)"=w160, "ClientID"=w157, "Broker IP"=w158) -> ()  [unwired: 8 in, 1 out]
          }
        }
        n151 = call-dynamic "Delacor_lib_QMH_Error Handler - Message Handling Loop.vi"("error in (no error)"=w143, "Message Queue in"=w145) -> ("dup error in"=w151:errorcluster)  [unwired: 8 in, 1 out]
      }
      n152 = while {
        shift-right: [w39] -> _
        shift-left: -1 -> [w38]
        tunnel: w22 -> [w36]
        shift-right: [w35] -> _
        shift-left: _ -> [w34]
        stop <- w37 stop-if-true
        # "Helper Loop"
        n153 = event shown="[0] Timeout" {
          selector: w36 -> [_ _ _ _]
          dyn-events: _ -> [_ _ _ _]
          timeout: w38 -> [_ _ _ _]
          tunnel: [w48 _ 10 -1] -> w39
          tunnel: w38 -> [w48 _ _ _]
          tunnel: [FALSE w66 _ _] -> w37
          tunnel: [w46 _ w68 w69] -> w35
          tunnel: w34 -> [w46 _ _ w69]
          event Timeout {
            n154 = event-data() -> ()  [unwired: 1 in, 1 out]
            n155 = call "MQTT_Read_Published_Message.vi"("connection ID"=w46) -> ("error out"=w45:errorcluster, "Message"=w43:string, "Topic Name"=w44:string)  [unwired: 5 in, 3 out]
            n156 = case shown="No Error" w45 {
              tunnel: w44 -> [w54 _]
              tunnel: w43 -> [w53 _]
              frame No Error {
                # "Sort message by topic"
                n157 = Match Pattern(string=w54, regular expression="/") -> (after substring=w55:string)  [unwired: 1 in, 3 out]
                n158 = case shown="\"False\", Default" w55 {
                  tunnel: w54 -> [w58 _]
                  tunnel: w53 -> [w57 w62]
                  frame "False", Default {
                    n159 = call "RX.vi"("Message"=w57, "Topic"=w58) -> ()  [unwired: 9 in, 1 out]
                  }
                  frame "HB" {
                    n160 = Tick Count (ms)() -> (millisecond timer value=w64:u32)
                    n161 = Scan From String(input string=w62, default 1=w64) -> (output 1=w65:u32)  [unwired: 3 in, 3 out]
                    n162 = Subtract(x=w64, y=w65) -> (x-y=→"Latency (ms)":u32)
                    n163 = feedback #2(u32 0 ("s? t:f")) -> (w60:u32)
                    n164 = Increment(x=w60) -> (x+1=w59:u32)
                    "HB RX Count" <- w59
                    n165 = feedback-in #2(w59) -> ()
                  }
                }
                "Rx Topic Name" <- w54
                "Rx Message" <- w53
              }
              frame Error {
              }
            }
            n166 = call "HB Timeout.vi"("HB Timeout ms"=u32 5000) -> ("Timeout"=w42:bool, "millisecond timer value"=w41:u32)  [unwired: 9 in]
            n167 = case shown="True" w42 {
              tunnel: w41 -> [_ w49]
              frame False {
              }
              frame True {
                n168 = call-poly "MQTT Message(poly).vi"() -> ()  [unwired: 11 in, 1 out]
                n169 = feedback #3(u32 0 ("s? t:f")) -> (w51:u32)
                n170 = Increment(x=w51) -> (x+1=w50:u32)
                "HB TX Count" <- w50
                n171 = feedback-in #3(w50) -> ()
                "ms" <- w49
              }
            }
          }
          event User Event {
            n172 = event-data() -> ("Exit"=w66:bool)  [unwired: 1 in, 4 out]
          }
          event User Event {
            # "Start listening to subscribed topics. Set ms timeout to 10 ms and pass TCP connecton refnum to shift register."
            n173 = event-data() -> ("MQTT Connection"=w68:refnum<k5>)  [unwired: 1 in]
          }
          event User Event {
            n174 = event-data() -> ()  [unwired: 1 in, 1 out]
          }
        }
      }
    }
    frame Error {
      # "Synchronize Caller Events.vi will inform Start Module.vi that the module has launched and will let the code calling Start Module.vi register for broadcasts and would permit the caller receive the broadcast that an error occurred at launch time."
      n175 = call "Synchronize Caller Events.vi"("Singleton Module Admin in"=w364) -> ("error out"=w369:errorcluster)  [unwired: 9 in, 1 out]
      n176 = call "Module Name--constant.vi"() -> ("Module Name"=w367:string)  [unwired: 11 in]
      n177 = Format Into String(format string="An error occurred during initialization. %s is no longer running.", w367) -> (resulting string=w365:string)  [unwired: 2 in, 1 out]
      n178 = Merge Errors(w371, w369) -> (w370:errorcluster)
      n179 = call "Error Reported.vi"("Additional Information"=w365, "Error"=w370) -> ()  [unwired: 9 in, 1 out]
    }
  }
  n180 = Merge Errors(w15, w18) -> (w14:errorcluster)
  n181 = call "Close Module.vi"("error in (no error)"=w14, "Module Admin in"=w9) -> ("error out"=w16:errorcluster, "External Launch"=w3:bool, "Module Admin out"=w4:refnum<class "Delacor_lib_QMH_Module Admin.lvclass">)  [unwired: 7 in]
  n182 = Unregister For Events(event registration refnum=w8, error in=w16) -> (error out=w13:errorcluster)
  "error out" <- w13
  n183 = case "External Launch?" shown="True" w3 {
    tunnel: w13 -> [_ w372]
    frame False {
    }
    frame True {
      n184 = case shown="No Error" w372 {
        frame No Error {
          n185 = invoke class="VI" method="FP.Close"() -> ()  [unwired: 3 in, 3 out]
        }
        frame Error {
          n186 = invoke class="VI" method="FP.Open"("Activate"=TRUE ("Activate?")) -> ()  [unwired: 4 in, 5 out]
        }
      }
    }
  }
  n187 = local write "Module Admin"(w4) -> ()
